vi "rangelimiter.vi"(8 "Upper lim":fxp<+/-,16,16>, 9 "Lower lim":fxp<+/-,16,16>, 11 "Input":fxp<+/-,16,16>) -> (3 "Output":fxp<+/-,16,16>)   [LabVIEW 2018]
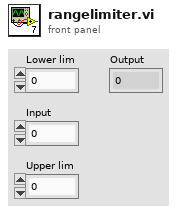
[diagram p1: front panel]
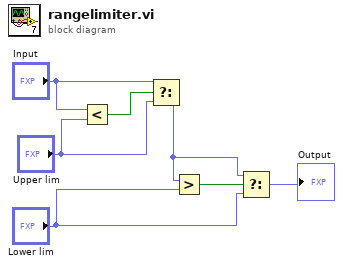
[diagram p0: block diagram]
diagram:
  n1 = Less?(x="Input", y="Upper lim") -> (x < y?=w7:bool)
  n2 = Select(t="Input", s=w7, f="Upper lim") -> (s? t:f=w3:fxp<+/-,16,16>)
  n3 = Greater?(x=w3, y="Lower lim") -> (0:w4:bool)
  n4 = Select(t=w3, s=w4, f="Lower lim") -> (s? t:f=→"Output":fxp<+/-,16,16>)
